vi "Check Shutter Rate.vi"(1 "Camera Settings":T1={"Exposure Time (ms)"=100.0, "Binning"=enum."2x2", "Scan Mode"=0, "Frames to Acquire"=1000.0, "Pixel Correction"=FALSE, "Frames to Skip"=0, "File Path"=path "", "Duty cycle"=0.0, "ALEX"=FALSE, "Shutter Enable"=[]} {"Exposure Time (ms)" min=1.0 max=10000.0 step=1.0}, 2 "Max rate (Hz)":dbl=20.0 format="%#_13g") -> (0 "Too fast?":bool)   [LabVIEW 2018, in "Synchronization Device.lvlib" / "Synchronization Device.lvclass"]
uses:
  Synchronization Device.lvclass
  Resources/Type Defs/Camera Settings.ctl
panel:
  in  "Stream Exposure Time":dbl=10.0 min=0.001 max=10000.0
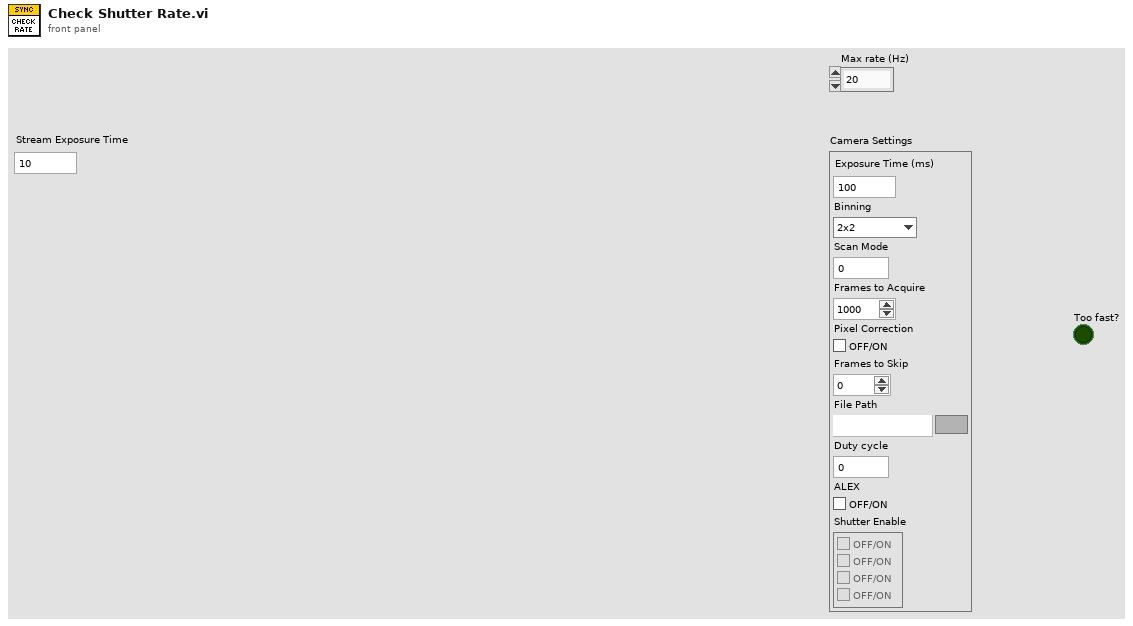
[diagram p1: front panel]
types:
  T1 = typedef "Camera Settings.ctl" = cluster{"Exposure Time (ms)":dbl, "Binning":enum16{"1x1", "2x2", "4x4"}, "Scan Mode":i32, "Frames to Acquire":dbl, "Pixel Correction":bool, "Frames to Skip":u32, "File Path":path, "Duty cycle":dbl, "ALEX":bool, "Shutter Enable":bool[]}
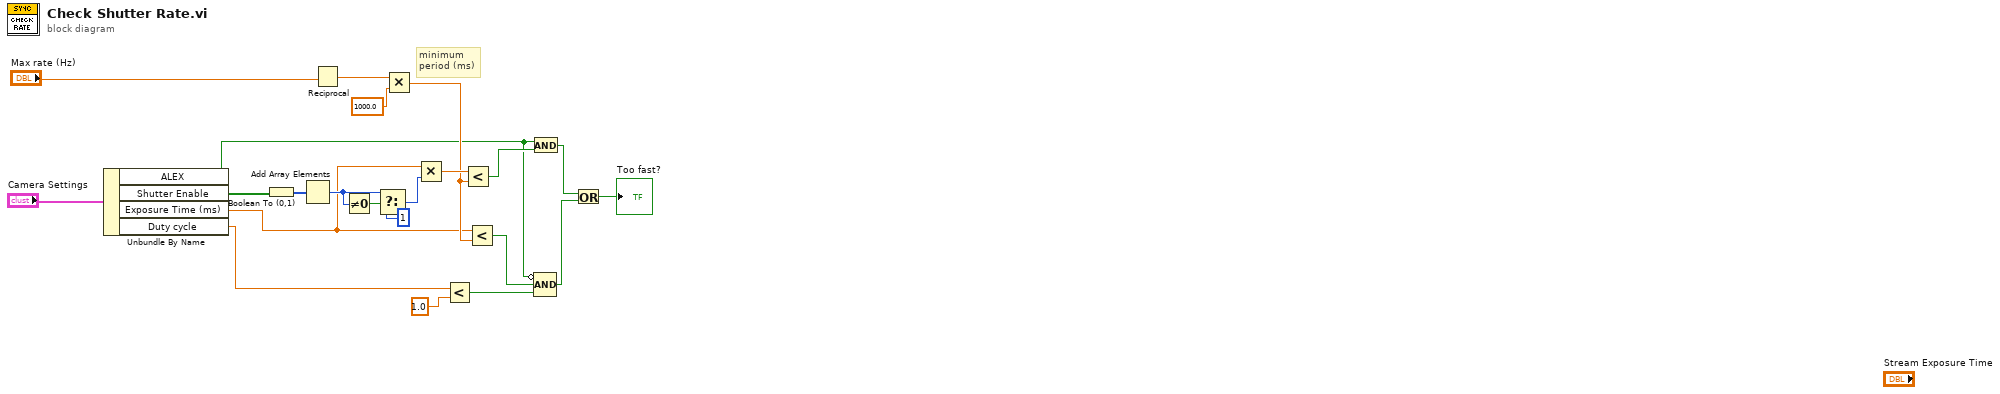
[diagram p0: block diagram]
diagram:
  # "minimum\nperiod (ms)"
  n1 = Unbundle By Name("Camera Settings") -> ("ALEX"=w5:bool, "Shutter Enable"=w4:bool[], "Exposure Time (ms)"=w3:dbl, "Duty cycle"=w2:dbl)
  n2 = Boolean To (0,1)(Boolean=w4) -> (0, 1=w11:i16[])
  n3 = Add Array Elements(numeric array=w11) -> (sum=w8:i16)
  n4 = Reciprocal(x="Max rate (Hz)") -> (1/x=w14:dbl)
  n5 = Not Equal To 0?(x=w8) -> (x != 0?=w9:bool)
  n6 = Select(t=w8, s=w9, f=i16 1) -> (s? t:f=w10:i16)
  n7 = Multiply(x=w14, y=1000.0) -> (x*y=w12:dbl)
  n8 = Multiply(x=w3, y=w10) -> (x*y=w22:dbl)
  n9 = Less?(x=w2, y=1.0) -> (x < y?=w18:bool)
  n10 = Less?(x=w22, y=w12) -> (x < y?=w19:bool)
  n11 = Less?(x=w3, y=w12) -> (x < y?=w16:bool)
  n12 = And(x=w5, y=w19) -> (x .and. y?=w21:bool)
  n13 = Compound Arithmetic op=AND(invert w5, w16, w18) -> (w17:bool)
  n14 = Or(x=w21, y=w17) -> (x .or. y?=→"Too fast?":bool)
